vi "Replace Scheduled Cell.vi"(8 "error in (no error)":errorcluster, 9 "Index":i32, 10 "Schedule Cell":refnum<class "Schedule Cell.lvclass">, 11 "Run Block in":refnum<class "Run Block.lvclass">) -> (0 "error out":errorcluster, 3 "Run Block out":refnum<class "Run Block.lvclass">)   [LabVIEW 2020, in "TALOS.lvlib" / "Run Utilities.lvlib" / "Run Block.lvclass"]
uses:
  Run Block.lvclass
  Cell/Schedule Cell.lvclass
  Run Block.lvclass/Run Block.ctl
  Schedule/Schedule.lvclass
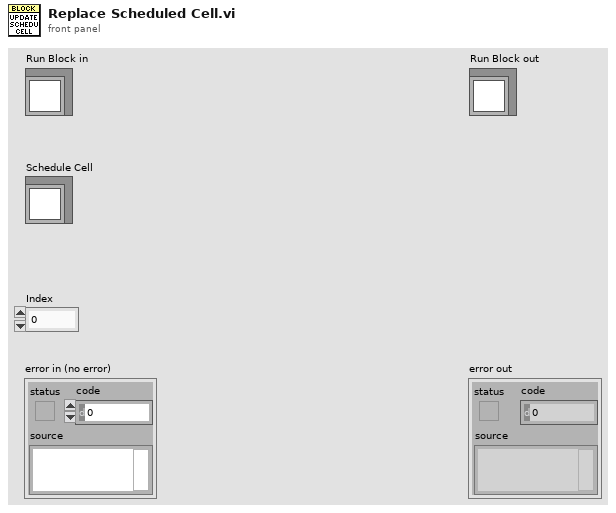
[diagram p1: front panel]
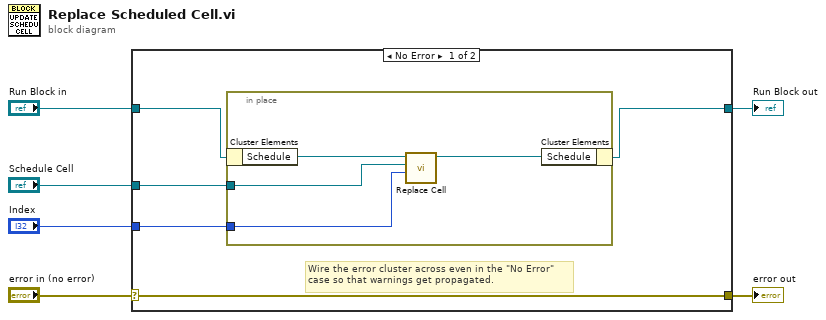
[diagram p0: block diagram]
diagram:
  n1 = case shown="No Error" "error in (no error)" {
    selector: "error in (no error)" -> [w11 w17]
    tunnel: [w11 w17] -> w5
    tunnel: [w7 w16] -> w3
    tunnel: "Run Block in" -> [w10 w16]
    tunnel: "Index" -> [w9 _]
    tunnel: "Schedule Cell" -> [w8 _]
    frame No Error {
      # "Wire the error cluster across even in the \"No Error\"\ncase so that warnings get propagated."
      n2 = in-place {
        in-place-border: w9 -> [w13]
        in-place-border: w8 -> [w12]
        n3 = in-place-cluster #1(w10) -> ("Schedule"=w15:refnum<class "Schedule.lvclass">)
        n4 = call-dynamic "Replace Cell.vi"("Index"=w13, "Schedule Cell"=w12, "Schedule in"=w15) -> ("Schedule out"=w14:refnum<class "Schedule.lvclass">)  [unwired: 7 in, 1 out]
        n5 = in-place-cluster #1("Schedule"=w14) -> (w7:refnum<class "Run Block.lvclass">)
      }
    }
    frame Error {
    }
  }
  "error out" <- w5
  "Run Block out" <- w3
